vi "Pin Test Utility.vi"() -> ()   [LabVIEW 2012]
uses:
  Type/_RT Command.ctl
  <vilib>/Utility/config.llb/Read Key (String).vi
  Configuration/_Global Configuration.vi
  <vilib>/Utility/config.llb/NI_LVConfig.lvlib
panel:
  in  "About":bool
  in  "PinState":bool
  out "Read Back":bool
  in  "Pin Address":u16 max=95 step=1
  in  "Read":bool
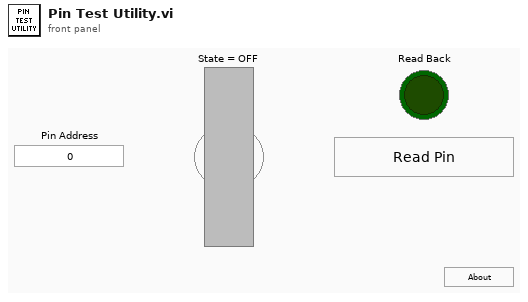
[diagram p1: front panel]
types:
  T1 = typedef "_RT Command.ctl" = enum16{"Start", "Stop", "Runtime Update", "Get Data", "Get Info", "Get Status", "Get Param", "Get Config", "Get Table", "Read ADC", "Set Oscillator", "Update Config", "Update Table", "Set All Pol", "Set Pol and DC", "Set Max Mass", "Toggle RP", "Toggle EL", "Set PIC", "Initialize Turbo", "Send Turbo Comm", "Close Turbo", "P1", "P2", "P3", "Send Serial", "Set LC Out", "Get LC In", "Read VAC", "Test Table", "Toggle Power", "Get Startup", "Set Startup", "Get ADC Table", "Set ADC Table", "Get Brief Status", "Get Detail Status", "Auxiliary Update", "Set CC Logics", "Set CC Input Logics", "Ignore Error"}
  T2 = typedef "NI_LVConfig.lvlib/Config Data RefNum.ctl" = refnum<k1>
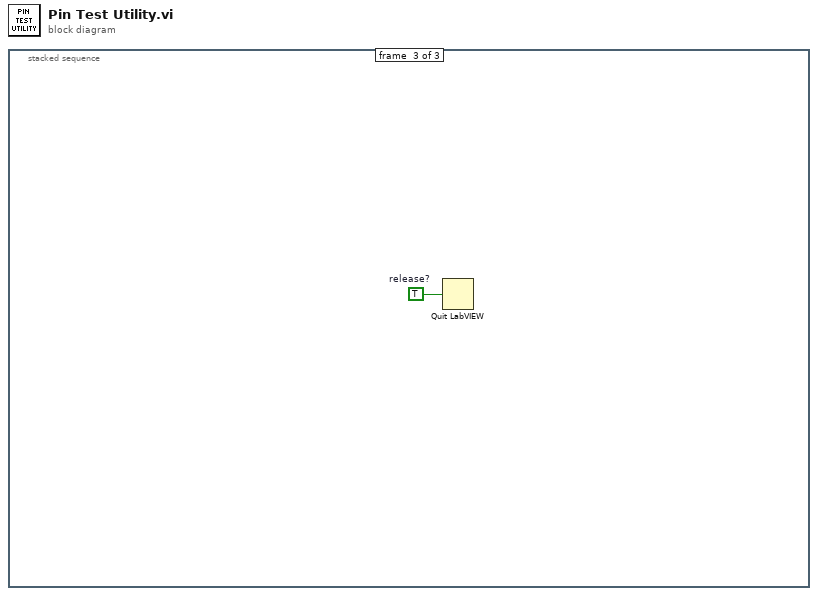
[diagram p0: block diagram]
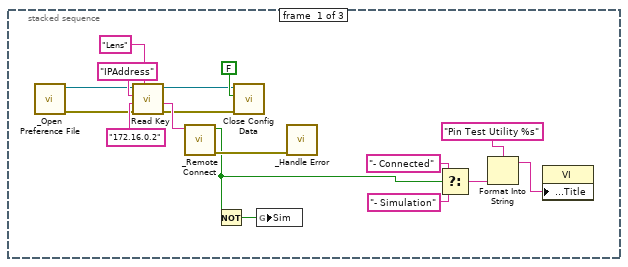
[diagram p2: hidden frame]
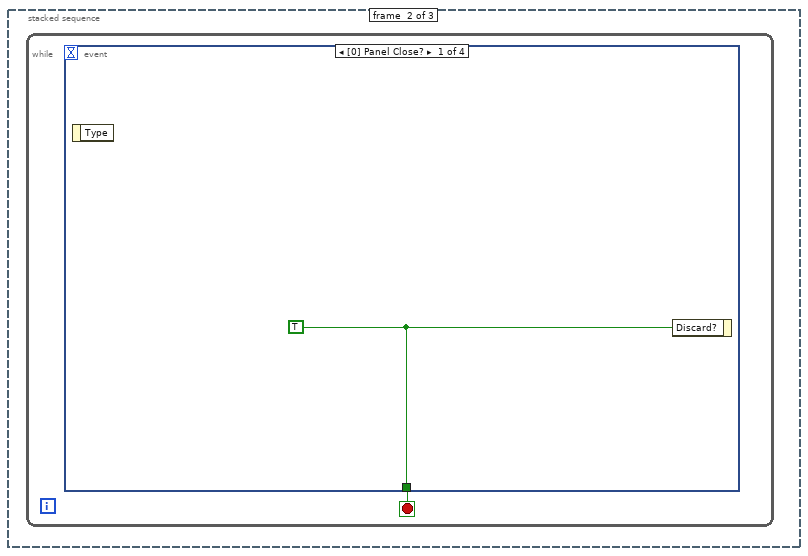
[diagram p3: hidden frame]
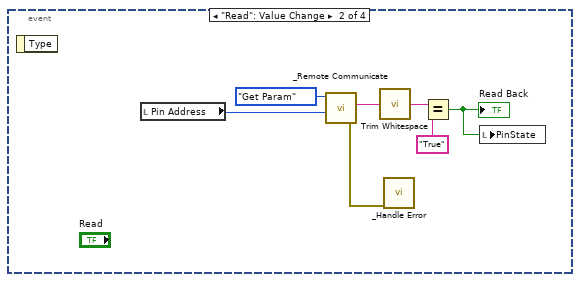
[diagram p4: hidden frame]
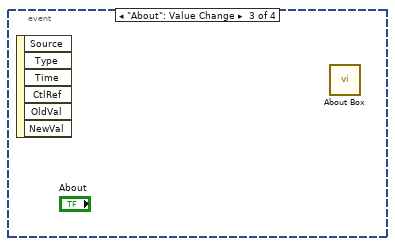
[diagram p5: hidden frame]
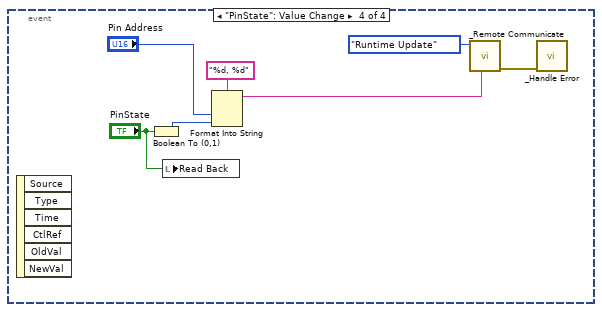
[diagram p6: hidden frame]
diagram:
  n1 = stacked-sequence {
    frame #0 {
      n2 = call "_Open Preference File.vi"() -> ("error"=w10:errorcluster, "refnum"=w11:T2)  [unwired: 1 in, 5 out]
      n3 = call-poly <vilib>:"Read Key.vi"("section"="Lens", "error in (no error)"=w10, "default value"="172.16.0.2", "key"="IPAddress" ("section"), "refnum"=w11) -> ("error out"=w8:errorcluster, "value"=w16:string, "refnum out"=w9:T2)  [unwired: 1 in, 3 out]
      n4 = call "_Remote Connect.vi"("IP Address"=w16) -> ("error out"=w7:errorcluster, "TCP"=w1:bool)  [unwired: 1 in, 4 out]
      n5 = Not(x=w1) -> (.not. x?=w15:bool)
      n6 = call <vilib>:"Close Config Data.vi"("error in (no error)"=w8, "write file if changed (T)"=FALSE ("write configuration file? (T)"), "refnum"=w9) -> ()  [unwired: 9 out]
      n7 = global write "_Global Configuration.vi" "Sim"(w15) -> ()
      n8 = call "_Handle Error.vi"("error in (no error)"=w7) -> ()  [unwired: 2 in, 5 out]
      n9 = Select(t="- Connected", s=w1, f="- Simulation") -> (s? t:f=w6:string)
      n10 = Format Into String(format string="Pin Test Utility %s", w6) -> (resulting string=w3:string)  [unwired: 2 in, 1 out]
      n11 = property class="VI"("Front Panel Window:Title"=w3) -> ()  [unwired: 2 in, 2 out]
    }
    frame #1 {
      n12 = while {
        stop <- w18 stop-if-true
        n13 = event shown="[0] Panel Close?" {
          selector: _ -> [_ _ _ _]
          dyn-events: _ -> [_ _ _ _]
          timeout: _ -> [_ _ _ _]
          tunnel: [w19 _ _ _] -> w18
          event Panel Close? {
            w19 = TRUE ("Discard?")
            n14 = event-data() -> ()  [unwired: 2 out]
            n15 = event-data("Discard?"=w19) -> ()  [unwired: 1 in, 1 out]
          }
          event "Read": Value Change {
            n16 = event-data() -> ()  [unwired: 2 out]
            n17 = local read "Pin Address"() -> (w25:u16)
            n18 = call "_Remote Communicate.vi"("DC Param"=w25, "Command"=_RT_Command."Get Param") -> ("error out"=w20:errorcluster, "Info"=w24:string)  [unwired: 4 in, 2 out]
            n19 = call <vilib>:"Trim Whitespace.vi"("string"=w24) -> ("trimmed string"=w23:string)  [unwired: 1 in]
            n20 = call "_Handle Error.vi"("error in (no error)"=w20) -> ()  [unwired: 2 in, 5 out]
            n21 = Equal?(x=w23, y="True") -> (x = y?=w21:bool)
            "Read Back" <- w21
            n22 = local write "PinState"(w21) -> ()
          }
          event "About": Value Change {
            n23 = event-data() -> ()  [unwired: 7 out]
            n24 = call "About Box.vi"() -> ()  [unwired: 1 out]
          }
          event "PinState": Value Change {
            n25 = event-data() -> ()  [unwired: 7 out]
            n26 = Boolean To (0,1)(Boolean="PinState") -> (0, 1=w31:i16)
            n27 = local write "Read Back"("PinState") -> ()
            n28 = Format Into String(format string="%d, %d", "Pin Address", w31) -> (resulting string=w29:string)  [unwired: 2 in, 1 out]
            n29 = call "_Remote Communicate.vi"("String"=w29, "Command"=_RT_Command."Runtime Update") -> ("error out"=w28:errorcluster)  [unwired: 4 in, 3 out]
            n30 = call "_Handle Error.vi"("error in (no error)"=w28) -> ()  [unwired: 2 in, 5 out]
          }
        }
      }
    }
    frame #2 {
      w34 = TRUE  # release?
      n31 = Quit LabVIEW(quit? (T)=w34) -> ()
    }
  }
